vi "Add Permissions.vi"(8 "error in (no error)":errorcluster, 9 "Accounts and Actions":T1[](array[typedef]), 10 "Label":string, 11 "SQS in":refnum<class "Queue.lvclass">) -> (0 "error out":errorcluster, 3 "SQS out":refnum<class "Queue.lvclass">)   [LabVIEW 2015, in "NI_AWS_SQS.lvlib" / "Queue.lvclass"]
doc: "Adds a permission to a queue for a specific principal. This allows sharing access to the queue.\n\nWhen you create a queue, you have full control access rights for the queue. Only you, the owner of the queue, can grant or deny permissions to the queue."
uses:
  Queue.lvclass
  Account and Action.ctl
  Permission Action.ctl
  Core/HTTP Request/Name Value Pair.ctl
  Core/HTTP Request/Request Options.ctl
  Core/HTTP Request/Region handling.ctl
  Core/HTTP Request/URL formatting.ctl
  Queue.lvclass/Queue.ctl
  Read Account Number.vi
  Read Name.vi
  Core/HTTP Request/HTTP Request.lvclass
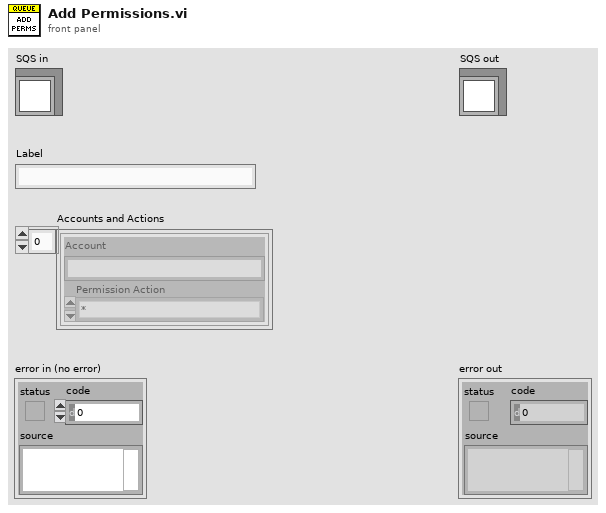
[diagram p1: front panel]
types:
  T1 = typedef "NI_AWS_SQS.lvlib/Queue.lvclass/Account and Action.ctl" = cluster{"Account":string, "Permission Action":T2}
  T2 = typedef "NI_AWS_SQS.lvlib/Queue.lvclass/Permission Action.ctl" = enum16{"*", "ChangeMessageVisibility", "DeleteMessage", "GetQueueAttributes", "GetQueueUrl", "ReceiveMessage", "SendMessage"}
  T3 = typedef "NI_AWS_Core.lvlib/HTTP Request.lvclass/Name Value Pair.ctl" = cluster{"name":string, "value":string}
  T4 = typedef "NI_AWS_Core.lvlib/HTTP Request.lvclass/Request Options.ctl" = cluster{"request headers":T3[], "request parameters":T3[], "request body":string, "region handling":T5, "URL formatting":T6}
  T5 = typedef "NI_AWS_Core.lvlib/HTTP Request.lvclass/Region handling.ctl" = enum16{"use region everywhere", "use region (authentication only)", "use region (URL only)", "ignore region everwhere"}
  T6 = typedef "NI_AWS_Core.lvlib/HTTP Request.lvclass/URL formatting.ctl" = enum16{"region-", "region."}
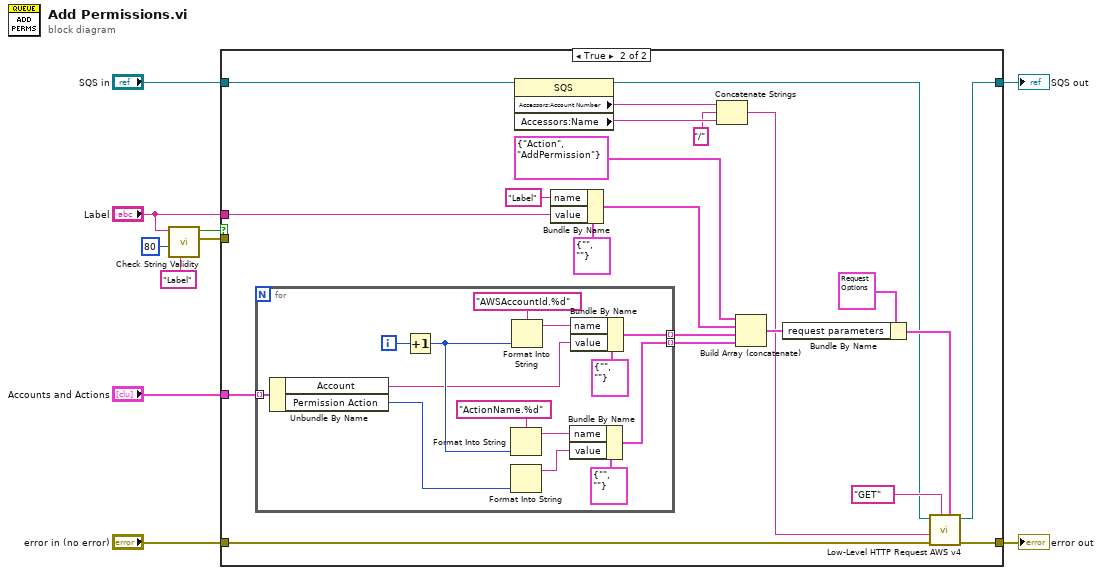
[diagram p0: block diagram]
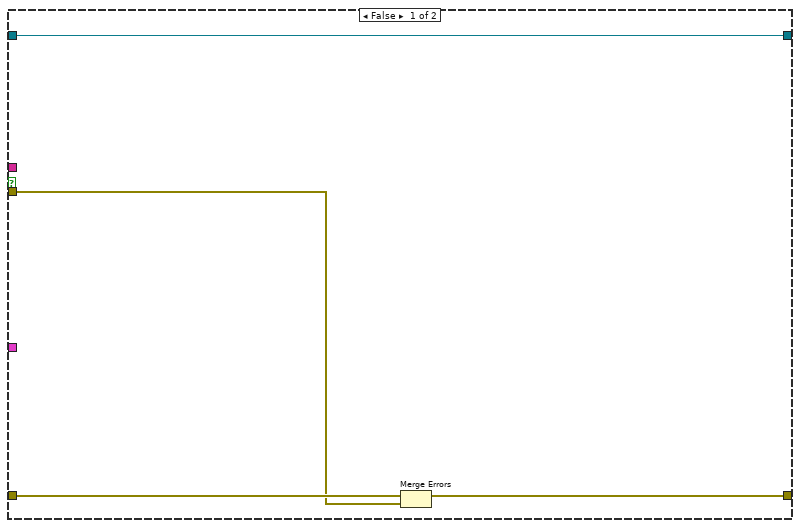
[diagram p2: hidden frame]
diagram:
  n1 = call "Check String Validity.vi"("String Name for Error"="Label", "Max Characters"=80, "String"="Label") -> ("string error"=w2:errorcluster, "Valid"=w3:bool)  [unwired: 7 in]
  n2 = case shown="True" w3 {
    tunnel: "SQS in" -> [w11 w28]
    tunnel: [w11 w15] -> w9
    tunnel: [w13 w27] -> w8
    tunnel: "error in (no error)" -> [w14 w26]
    tunnel: "Accounts and Actions" -> [_ w25]
    tunnel: "Label" -> [_ w19]
    tunnel: w2 -> [w12 _]
    frame False {
      n3 = Merge Errors(w14, w12) -> (w13:errorcluster)
    }
    frame True {
      n4 = for {
        tunnel: w25 -> [w44] mode=indexing
        tunnel: [w45] -> w33 mode=indexing
        tunnel: [w40] -> w29 mode=indexing
        i -> [w49]
        n5 = Unbundle By Name(w44) -> ("Account"=w38:string, "Permission Action"=w37:T2)
        n6 = Increment(x=w49) -> (x+1=w39:i32)
        n7 = Format Into String(format string="ActionName.%d", w39) -> (resulting string=w43:string)  [unwired: 2 in, 1 out]
        n8 = Format Into String(w37) -> (resulting string=w36:string)  [unwired: 3 in, 1 out]
        n9 = Format Into String(format string="AWSAccountId.%d", w39) -> (resulting string=w46:string)  [unwired: 2 in, 1 out]
        n10 = Bundle By Name(cluster=T3 {"name"="", "value"=""} ("element"), "name"=w43, "value"=w36) -> (w40:T3)
        n11 = Bundle By Name(cluster=T3 {"name"="", "value"=""} ("element"), "name"=w46, "value"=w38) -> (w45:T3)
      }
      n12 = property class="SQS"(reference=w28) -> (reference out=w16:refnum<class "Queue.lvclass">, "Accessors:Account Number"=w32:string, "Accessors:Name"=w31:string)  [unwired: 1 in, 1 out]
      n13 = Bundle By Name(cluster=T3 {"name"="", "value"=""} ("element"), "name"="Label", "value"=w19) -> (w21:T3)
      n14 = Concatenate Strings(w32, "/", w31) -> (w24:string)
      n15 = Build Array (concatenate)(T3 {"name"="Action", "value"="AddPermission"} ("Cluster"), w21, w33, w29) -> (w34:T3[])
      n16 = Bundle By Name(cluster=T4 {"request headers"=[], "request parameters"=[{"name"="Action", "value"="ListQueues"}], "request body"="", "region handling"=enum."use region everywhere", "URL formatting"=enum."region."} ("Request Options"), "request parameters"=w34) -> (w17:T4)
      n17 = call "Low-Level HTTP Request AWS v4.vi"("Request Options"=w17, "HTTP-Verb"="GET", "error in (no error)"=w26, "URL Suffix"=w24, "AWS Core in"=w16) -> ("error out"=w27:errorcluster, "AWS Core out"=w15:refnum<class "Queue.lvclass">)  [unwired: 3 in, 2 out]
    }
  }
  "error out" <- w8
  "SQS out" <- w9
